vi "Unregister.vi"(8 "error in (no error)":errorcluster) -> (0 "error out":errorcluster)   [LabVIEW 2019, in "FootScan Engine.lvlib"]
uses:
  FootScan Engine.lvlib
panel:
  # "Input"
  # "Output"
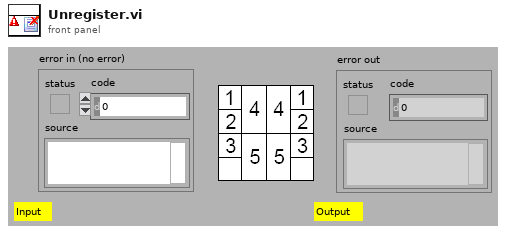
[diagram p1: front panel]
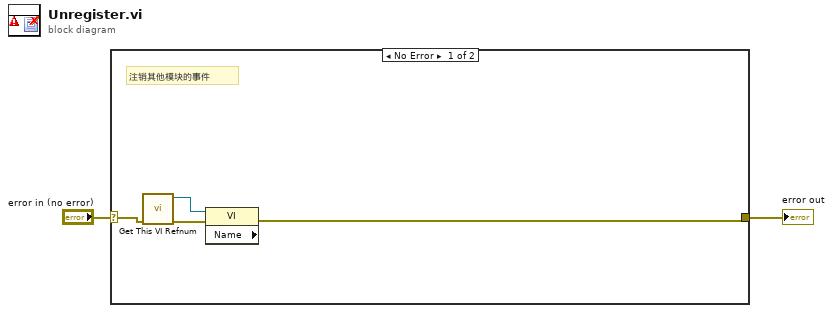
[diagram p0: block diagram]
diagram:
  n1 = case shown="No Error" "error in (no error)" {
    selector: "error in (no error)" -> [w5 w7]
    tunnel: [w3 w7] -> w1
    frame No Error {
      # "注销其他模块的事件"
      n2 = call "Get This VI Refnum.vi"("error in (no error)"=w5) -> ("error out"=w4:errorcluster, "This VI Refnum Out"=w6:refnum<vi>)  [unwired: 9 in]
      n3 = property class="VI" props=["Name"](reference=w6, error in=w4) -> (error out=w3:errorcluster)  [unwired: 2 out]
    }
    frame Error {
    }
  }
  "error out" <- w1
